vi "GPS PPS Syncronisation.vi"() -> ()   [LabVIEW 2015]
doc: "This template is for the Simple NI-USRP Streaming design, a design that shows the basics of streaming data to and from an NI USRP-294x/295x device. Refer to the block diagram for more information about how to use this template."
uses:
  <instrlib>/niUsrpRio/Config/v1/Host/Public/What to Query for.ctl
  Supporting Files/PPS Source.ctl
  <vilib>/userdefined/Silver/nirio_resource_slv.ctl
  SubVIs/Start Trigger.ctl
  <instrlib>/_niInstr/Register Bus/v0/Host/Public/Register Read Request.ctl
  <instrlib>/niUsrpRio/Config/v1/Host/Private/DB Types.ctl
  <vilib>/Utility/error.llb/DialogType.ctl
  PPS_Global_Var.vi
  Supporting Files/test_sup.vi
  <instrlib>/niUsrpRio/Config/v1/Host/niUsrpRio Config v1 Host.lvlib
  <instrlib>/_niInstr/Register Bus/v0/Host/niInstr Register Bus v0 Host.lvlib
panel:
  out "DaughterB":T1 caption="Daughter Board Name"
  in  "Tab Control 2":enum32{"XY Plot", "Coerced Config"}(tab)
  out "String 2":string
  out "XY Graph":cluster{i32[], dbl[]}[](graph)
  out "generating":bool caption="Generating"
  in  "tx.stop":bool
  out "tx.coerced configurations":T2
  in  "Tab Control":T3(tab)
  out "String":string
  out "PPS Pulse":bool
  in  "?":bool
  out "GPS Lock":bool
  in  "scope":string
  in  "What to Query for":T4=enum."GPS Lock Status"
  in  "PPS Source":T5=enum."gps pps"
  in  "Wait for GPS Lock?":bool=TRUE
  out "Minutes Elapsed (GPS Lock)":dbl
  in  "USRP RIO device":T6="RIO0" caption="USRP RIO Device"
  in  "Which Bitfile":string(combo)="Time"
  in  "Transmitter Config":T8={"rf enable 0"=TRUE, "rf config 0"={"antenna"="TX1", "frequency"=2000000000.0, "lo frequency"=-1.0, "level"=0.0}, "rf enable 1"=FALSE, "rf config 1"={"antenna"="TX1", "frequency"=2000000000.0, "lo frequency"=-1.0, "level"=0.0}, "transfer mode"=enum."Finite", "sample rate"=10000000.0, "number of samples"=8192, "start trigger"=enum."Immediate", "tone frequency"=100000.0} {"tone frequency" format="%#.3pHz"; "sample rate" format="%#.3pS/s"; "rf config 0"."level" format="%#_gdBm"; "rf config 0"."lo frequency" format="%#.3pHz"; "rf config 0"."frequency" format="%#.3pHz"; "rf config 1"."level" format="%#_gdBm"; "rf config 1"."lo frequency" format="%#.3pHz"; "rf config 1"."frequency" format="%#.3pHz"}
  out "RtmLog":string
  out "Error String":string
  in  "Debug":enum32{"Page 1", "Page 2"}(tab)
  out "GPSDO Stability Delay":bool
  out "FPGA Interface Open":bool
  out "USRP Session Status":bool
  out "Executing on FPGA":bool
  out "Target Adr.":T9 {"subsystem" format="%b"; "address" format="%.0b"}
  out "FPGA IO A":bool
  out "Halt: 2":bool
  out "Halt: 1":bool
  out "GPS Lock 2":bool
  out "TKeep Lock":bool
  out "PPS Stable":bool
  out "TkPSP":bool
  out "Which Target?":string
  in  "Interface Method":T10(ring)=enum."Open Dynamic Bitfile"
  out "Time Elapsed":string
  out "FPGA Version":dbl
  out "RIO Version":dbl
  out "Data Clock Rate":dbl
  out "Dautr Clock Rate":dbl
  out "FPGA Interface":dbl
  out "FPGA Board Ver.":dbl
  out "Status":dbl
  in  "Color Box":u32(colorbox)=11842740
  # "Overview"
  # "Aditional Config"
  # "Transmitter Config"
  # "Runtime Log Panel"
  # "Current Errors"
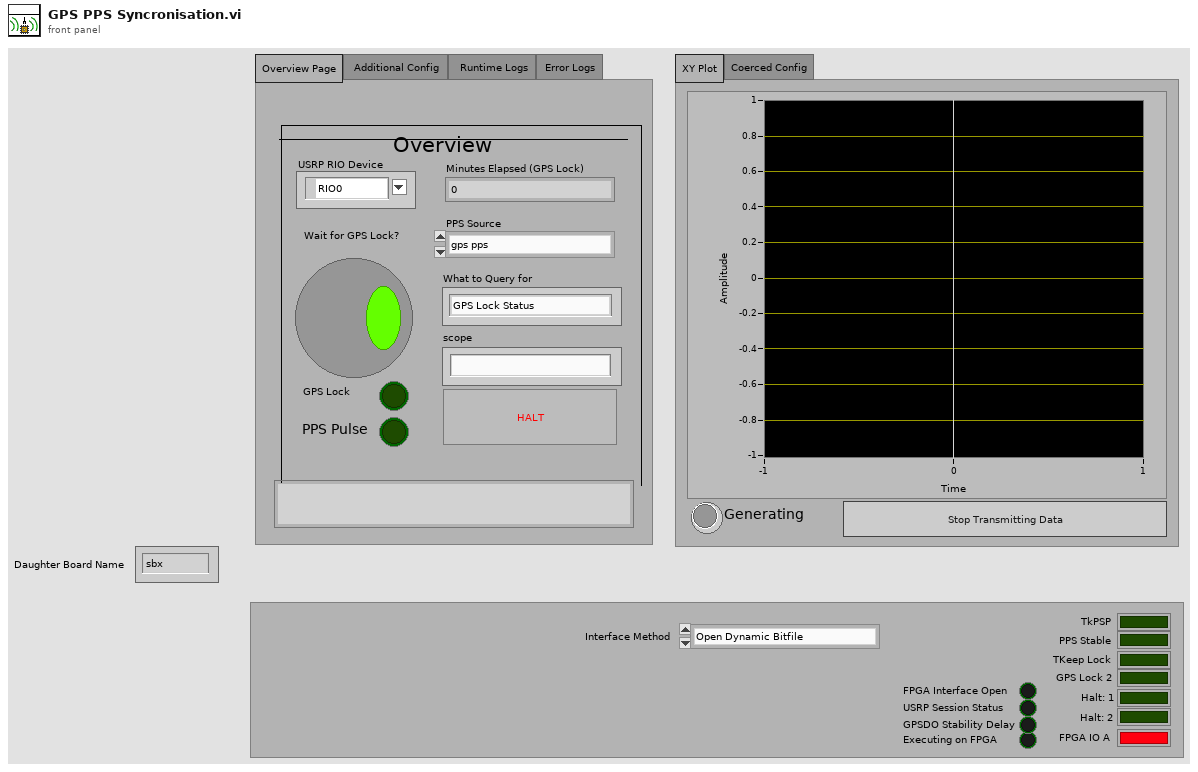
[diagram p1: front panel]
types:
  T1 = typedef "niUsrpRio Config v1 Host.lvlib/DB Types.ctl" = enum16{"sbx", "cbx", "wbx", "unknown"}
  T2 = cluster{"coerced frequencies":dbl[], "coerced lo frequencies":dbl[], "coerced levels":dbl[], "coerced sample rates":dbl[]}
  T3 = enum32{"Overview Page", " Additional Config ", " Runtime Logs ", "Error Logs "}
  T4 = typedef "niUsrpRio Config v1 Host.lvlib/What to Query for.ctl" = enum16{"Clock Chip Lock Status", "Clock Chip Ever Unlocked", "LO Lock Status", "GPS Lock Status", "GPS Ever Unlocked", "DRAM Ready Status", "DAC PLL Lock Status", "DAC Sync Lock Status", "Data Clock PLL Lock Status", "Data Clock PLL Ever Unlocked", "ADC Clock PLL Lock Status", "ADC Clock PLL Ever Unlocked", "ADC Data Valid Status", "ADC Data Ever Invalid"}
  T5 = typedef "PPS Source.ctl" = enum16{"external pps", "gps pps", "internal pps"}
  T6 = typedef "nirio_resource_slv.ctl" = tag
  T7 = typedef "Start Trigger.ctl" = enum8{"Software", "Digital Edge", "Rx Start Trigger", "Tx Start Trigger", "Immediate", "Future Time Event"}
  T8 = cluster{"rf enable 0":bool, "rf config 0":cluster{"antenna":string, "frequency":dbl, "lo frequency":dbl, "level":dbl}, "rf enable 1":bool, "rf config 1":cluster{"antenna":string, "frequency":dbl, "lo frequency":dbl, "level":dbl}, "transfer mode":enum16{"Finite", "Continuous"}, "sample rate":dbl, "number of samples":u32, "start trigger":T7, "tone frequency":dbl}
  T9 = typedef "niInstr Register Bus v0 Host.lvlib/Register Read Request.ctl" = cluster{"subsystem":u8, "address":u16}
  T10 = enum16{"Open FPGA", "Open Dynamic Bitfile", "Daisy Chain"}
  T11 = cluster{"tx config":cluster{"rf enable 0":bool, "rf config 0":cluster{"antenna":string, "frequency":dbl, "lo frequency":dbl, "level":dbl}, "rf enable 1":bool, "rf config 1":cluster{"antenna":string, "frequency":dbl, "lo frequency":dbl, "level":dbl}, "transfer mode":enum16{"Finite", "Continuous"}, "sample rate":dbl, "number of samples":u32, "start trigger":T7, "tone frequency":dbl}, "reference frequency source":string, "tx.enabled channels":string[], "I":i16[], "Q":i16[], "tx.coerced configurations":cluster{"coerced frequencies":dbl[], "coerced lo frequencies":dbl[], "coerced levels":dbl[], "coerced sample rates":dbl[]}}
  T12 = typedef "niUsrpRio Config v1 Host.lvlib/niUsrpRio Session.ctl" = cluster{"FPGA Interface":refnum<k20>, "RIO Interface Number":u32, "Data Clock Rate":u32, "FPGA Data Clock Rate":u32, "Global Settings Register Bus":T13, "Radio 0 Settings Register Bus":T13, "Radio 1 Settings Register Bus":T13, "Radio Settings Bus Semaphore":T14, "DB Queues":T15[], "Characterization Data Valid?":bool, "EEPROM Header":T16, "Device Data Header":T17, "EEPROM Characterization Header":T18, "Characterization Data":T19[], "FPGA Current Version":u32, "FPGA Oldest Compatible Version":u32, "Fixed Logic Current Version":u32, "Fixed Logic Oldest Compatible Version":u32, "FPGA Radio Settings Bus Current Version":u32, "FPGA Radio Settings Bus Oldest Compatible Version":u32, "FPGA Board Config Current Version":u32, "FPGA Board Config Oldest Compatible Version":u32}
  T13 = typedef "niInstr Register Bus v0 Host.lvlib/Register Bus Session.ctl" = refnum<queue>
  T14 = typedef "Semaphore RefNum" = refnum<k1>
  T15 = typedef "niUsrpRio Config v1 Host.lvlib/DB Queue Reference.ctl" = refnum<queue>
  T16 = typedef "niUsrpRio Config v1 Host.lvlib/EEPROM Header.ctl" = cluster{"Checksum":u32, "Product Code":u16, "Hardware Current Version":u16, "Hardware Oldest Compatible Version":u16, "EEPROM Map Current Version":u16, "EEPROM Map Oldest Compatible Version":u16, "User Password":string, "Pointer to Factory Header":u32, "Pointer to User Header":u32, "Recommended Interval":u16, "Number of Reserved Bytes":i32, "Number of Daughterboards":u8, "Daughterboard IDs":u16[], "Daughterboard Serial Numbers":string[]}
  T17 = typedef "niUsrpRio Config v1 Host.lvlib/EEPROM Device Data Header.ctl" = cluster{"Checksum":u32, "Number of Channels":u8, "Number of Gain Settings":u16[], "Pointer to Characterization Data":u32[], "Number of Reserved Bytes":i32, "Number of Frequencies":u16[]}
  T18 = typedef "niUsrpRio Config v1 Host.lvlib/EEPROM Characterization Header.ctl" = cluster{"Checksum":u32, "Date":timestamp, "Temperature":sgl, "Misc. Info":string, "Pointer to Device Data Header":u32, "Number of Reserved Bytes":i32}
  T19 = typedef "niUsrpRio Config v1 Host.lvlib/Characterization Data.ctl" = cluster{"Gains[dB]":dbl[], "Frequencies [Hz]":dbl[], "IQ Imbalance Table":T20[], "Measured Gains[dB]":dbl[][]}
  T20 = typedef "niUsrpRio Config v1 Host.lvlib/IQ Imbalance.ctl" = cluster{"Gain Imbalance [linear]":dbl, "Phase Imbalance [radians]":dbl, "Offset":cdb}
  T21 = typedef "DialogType.ctl" = u16
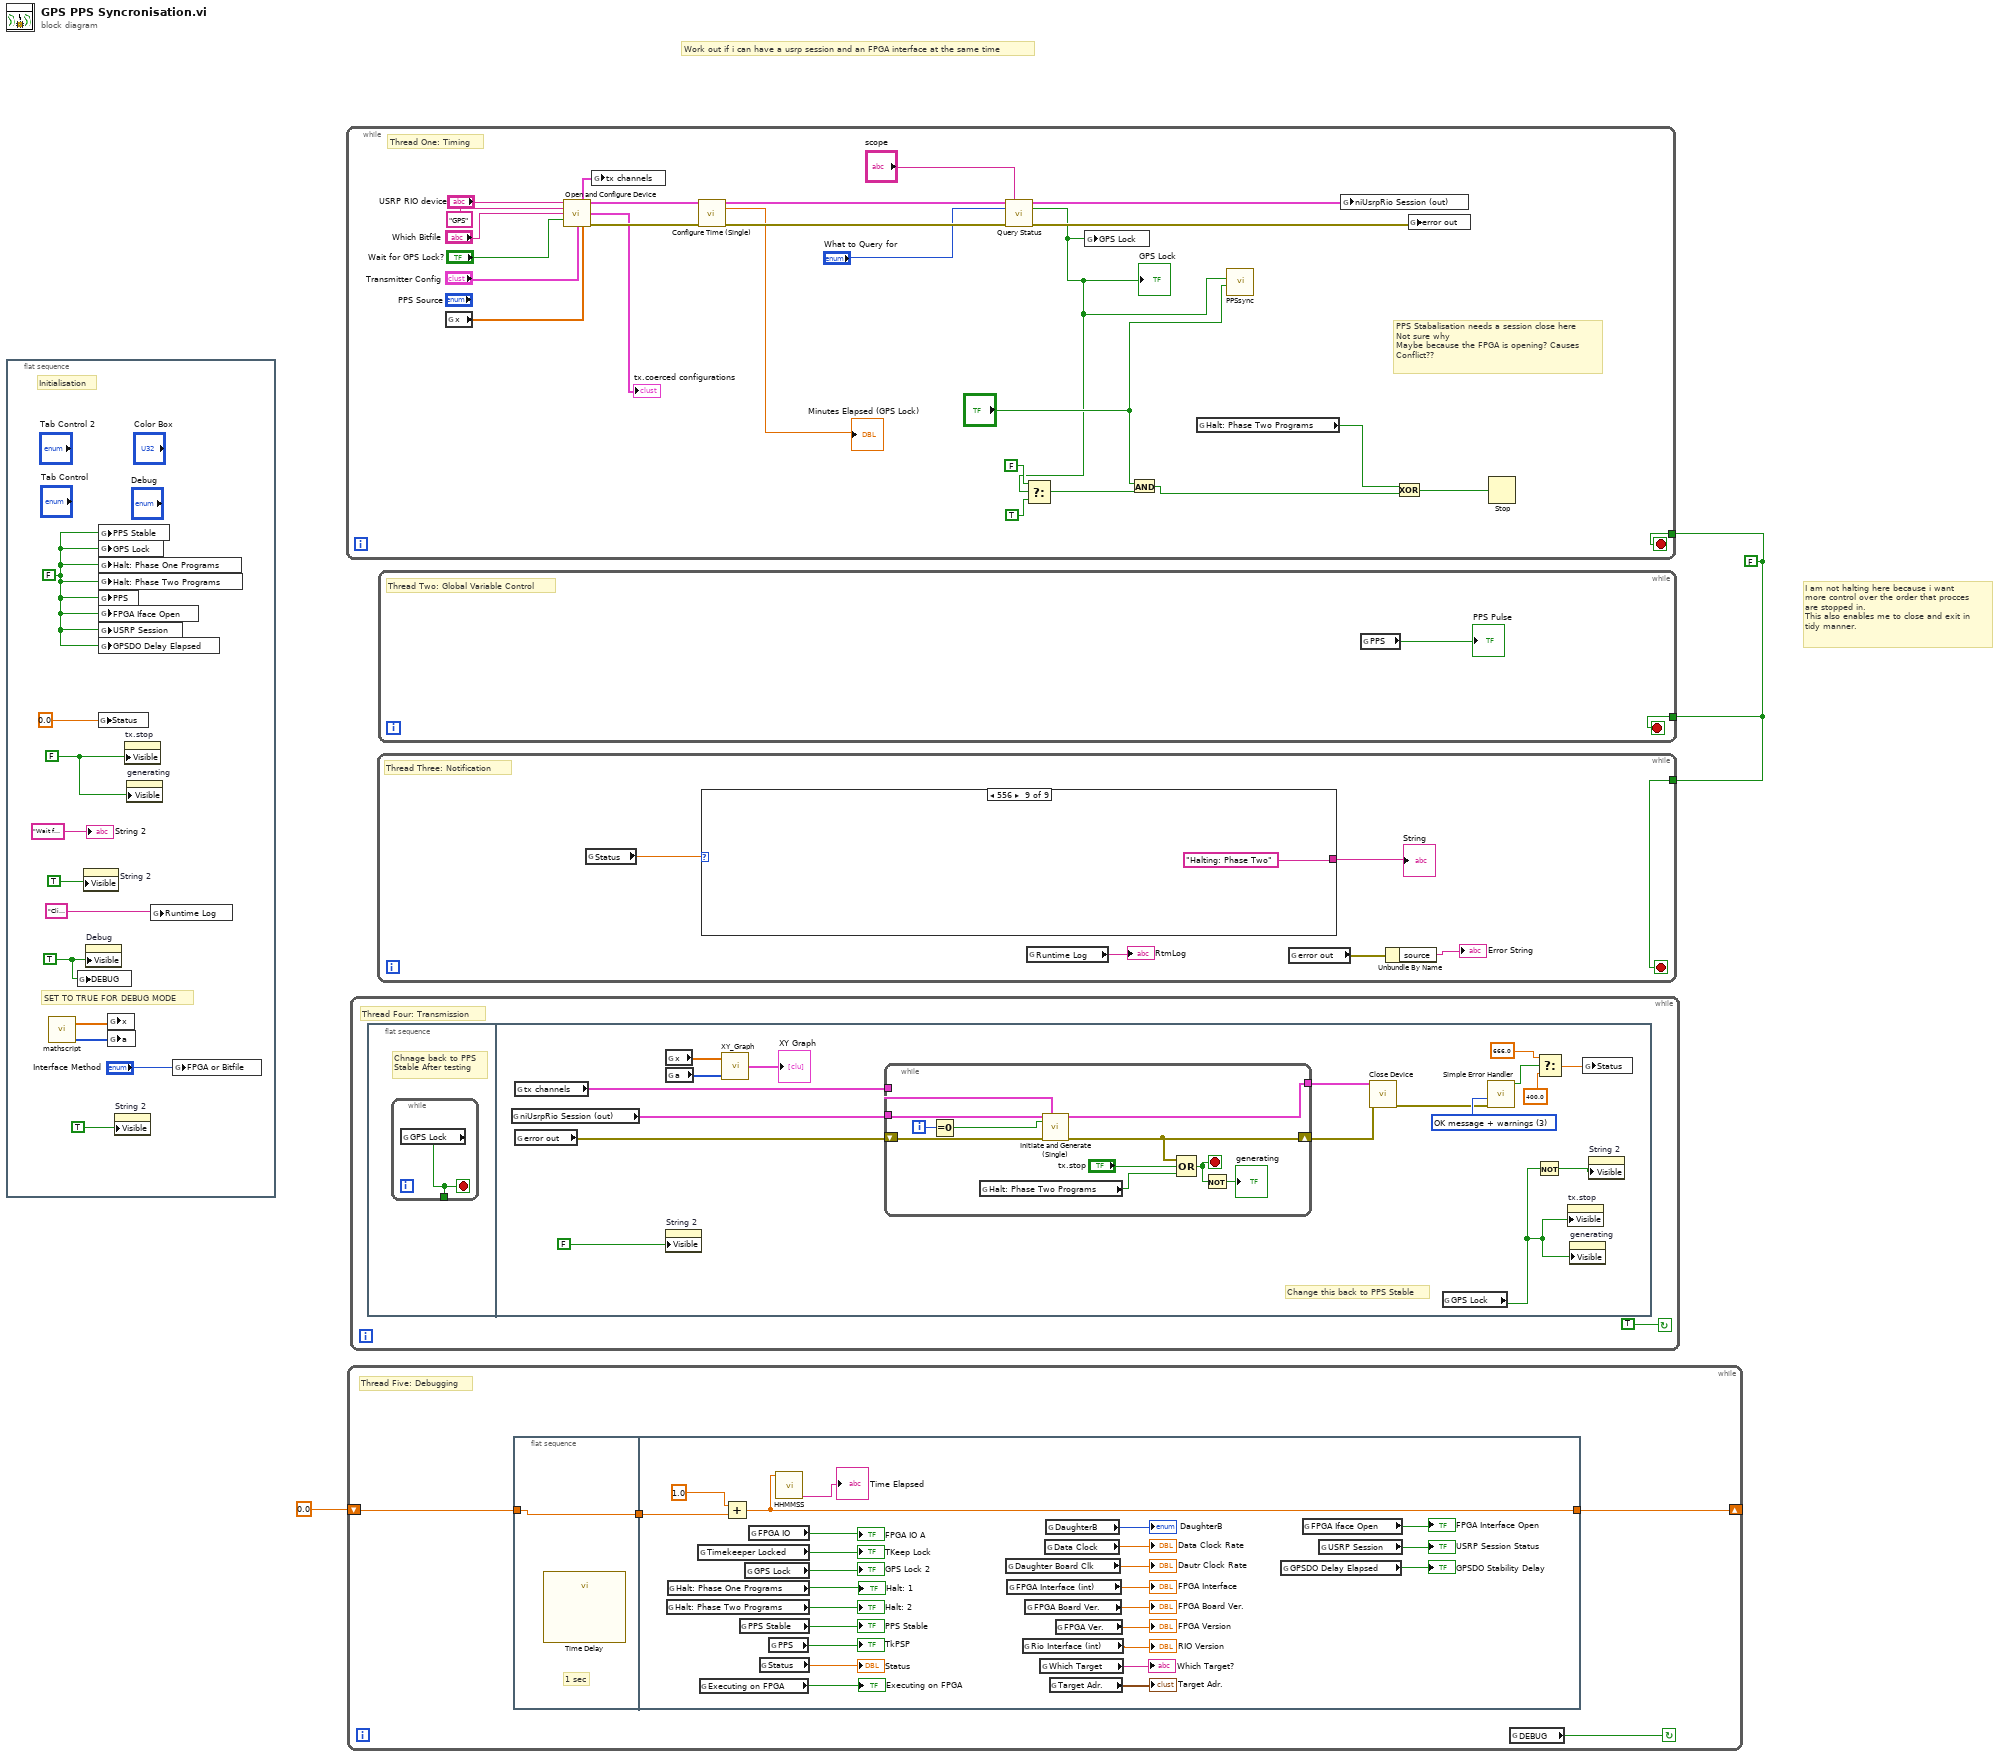
[diagram p0: block diagram]
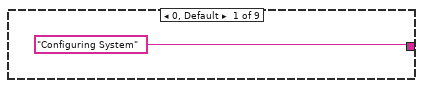
[diagram p2: hidden frame]
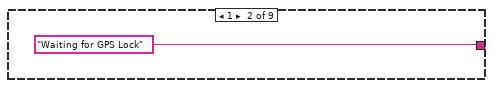
[diagram p3: hidden frame]
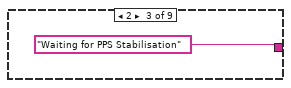
[diagram p4: hidden frame]
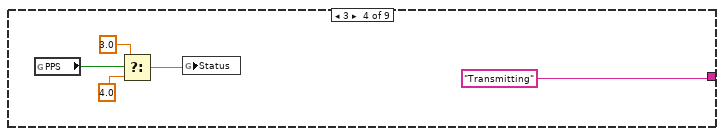
[diagram p5: hidden frame]
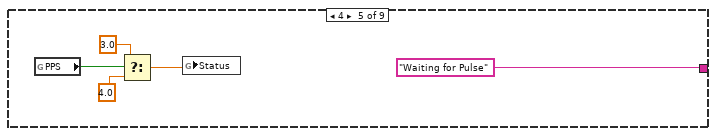
[diagram p6: hidden frame]
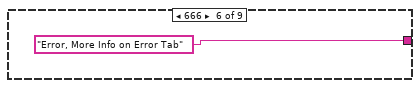
[diagram p7: hidden frame]
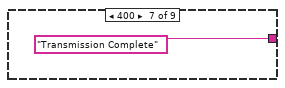
[diagram p8: hidden frame]
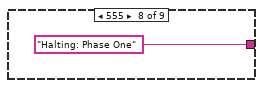
[diagram p9: hidden frame]
diagram:
  w2 = FALSE
  # "Work out if i can have a usrp session and an FPGA interface at the same time"
  # "I am not halting here because i want\nmore control over the order that procces\nare stopped in.\nThis also enables me to close and exit in \ntidy manner."
  n1 = flat-sequence {
    frame #0 {
      w7 = TRUE
      w8 = FALSE
      w5 = FALSE
      # "SET TO TRUE FOR DEBUG MODE"
      # "Initialisation"
      n2 = call "mathscript.vi"() -> ("a"=w11:enum16{""}[], "x"=w12:dbl[])  [unwired: 2 in]
      n3 = global write "PPS_Global_Var.vi" "DEBUG"(w7) -> ()
      n4 = property on="String 2" class="Str"("Visible"=TRUE) -> ()  [unwired: 2 in, 2 out]
      n5 = property on="Debug" class="TabCtl (strict)"("Visible"=w7) -> ()  [unwired: 2 in, 2 out]
      n6 = global write "PPS_Global_Var.vi" "Status"(0.0) -> ()
      n7 = global write "PPS_Global_Var.vi" "PPS Stable"(w5) -> ()
      n8 = global write "PPS_Global_Var.vi" "GPS Lock"(w5) -> ()
      n9 = global write "PPS_Global_Var.vi" "Halt: Phase One Programs"(w5) -> ()
      n10 = global write "PPS_Global_Var.vi" "Halt: Phase Two Programs"(w5) -> ()
      n11 = global write "PPS_Global_Var.vi" "PPS"(w5) -> ()
      n12 = global write "PPS_Global_Var.vi" "FPGA Iface Open"(w5) -> ()
      n13 = global write "PPS_Global_Var.vi" "USRP Session"(w5) -> ()
      n14 = global write "PPS_Global_Var.vi" "GPSDO Delay Elapsed"(w5) -> ()
      n15 = global write "PPS_Global_Var.vi" "x"(w12) -> ()
      n16 = global write "PPS_Global_Var.vi" "a"(w11) -> ()
      n17 = property on="String 2" class="Str"("Visible"=TRUE) -> ()  [unwired: 2 in, 2 out]
      n18 = property on="tx.stop" class="Bool"("Visible"=w8) -> ()  [unwired: 2 in, 2 out]
      n19 = property on="generating" class="Bool (strict)"("Visible"=w8) -> ()  [unwired: 2 in, 2 out]
      n20 = global write "PPS_Global_Var.vi" "Runtime Log"("ClickRun to to Begin") -> ()
      n21 = global write "PPS_Global_Var.vi" "FPGA or Bitfile"("Interface Method") -> ()
      "String 2" <- "Wait for GPS Lock before Transmission Can Begin"
    }
  }
  n22 = while {
    tunnel: w2 -> [w29]
    stop <- w29 stop-if-true
    # "PPS Stabalisation needs a session close here\nNot sure why\nMaybe because the FPGA is opening? Causes\nConflict??"
    # "Thread One: Timing"
    n23 = global read "PPS_Global_Var.vi" "x"() -> (w17:cdb[])
    n24 = call "Open and Configure Device.vi"("USRP RIO Device"="USRP RIO device", "reference frequency source"="GPS", "which bitfile"="Which Bitfile", "Wait for GPS Lock?"="Wait for GPS Lock?", "tx config"="Transmitter Config", "x"=w17) -> ("tx channels"=w18:T11, "niUsrpRio Session (out)"=w38:T12, "tx.coerced configurations"=→"tx.coerced configurations":T2, "error out"=w39:errorcluster)  [unwired: 3 in, 3 out]
    n25 = global write "PPS_Global_Var.vi" "tx channels"(w18) -> ()
    n26 = call "Configure Time (Single).vi"("niUsrpRio Session"=w38, "error in"=w39) -> ("niUsrpRio Session (out)"=w35:T12, "time elapsed"=→"Minutes Elapsed (GPS Lock)":dbl, "error out"=w36:errorcluster)  [unwired: 11 in]
    n27 = call <instrlib>:"Query Status.vi"("niUsrpRio Session"=w35, "scope"="scope", "What to Query for"="What to Query for", "error in"=w36) -> ("niUsrpRio Session (out)"=w16:T12, "Status"=w14:bool, "error out"=w15:errorcluster)  [unwired: 9 in]
    "GPS Lock" <- w14
    n28 = Select(t=FALSE, s=w14, f=TRUE) -> (s? t:f=w32:bool)
    n29 = global write "PPS_Global_Var.vi" "GPS Lock"(w14) -> ()
    n30 = And(x="?", y=w32) -> (x .and. y?=w30:bool)
    n31 = global read "PPS_Global_Var.vi" "Halt: Phase Two Programs"() -> (w28:bool)
    n32 = call "PPSsync.vi"("Halt"="?", "Advance"=w14) -> ()  [unwired: 4 in, 2 out]
    n33 = global write "PPS_Global_Var.vi" "niUsrpRio Session (out)"(w16) -> ()
    n34 = Exclusive Or(1:w30, 2:w28) -> (0:w31:bool)
    n35 = global write "PPS_Global_Var.vi" "error out"(w15) -> ()
    n36 = Stop(stop? (T)=w31) -> ()
  }
  n37 = while {
    shift-right: [w42] -> _
    shift-left: 0.0 -> [w41]
    stop <- w43 continue-if-true
    # "Thread Five: Debugging"
    n38 = flat-sequence {
      tunnel: w41 -> [w44]
      tunnel: [w44] -> w40
      tunnel: [w54] -> w42
      tunnel: w40 -> [w68]
      frame #0 {
        # "1 sec"
        n39 = call "Time Delay"() -> ()  [unwired: 11 in, 1 out]
      }
      frame #1 {
        n40 = global read "PPS_Global_Var.vi" "Halt: Phase Two Programs"() -> (→"Halt: 2":bool)
        n41 = global read "PPS_Global_Var.vi" "Halt: Phase One Programs"() -> (→"Halt: 1":bool)
        n42 = global read "test_sup.vi" "Timekeeper Locked"() -> (→"TKeep Lock":bool)
        n43 = global read "PPS_Global_Var.vi" "Executing on FPGA"() -> (→"Executing on FPGA":bool)
        n44 = Add(x=1.0, y=w68) -> (x+y=w54:dbl)
        n45 = global read "PPS_Global_Var.vi" "PPS Stable"() -> (→"PPS Stable":bool)
        n46 = global read "PPS_Global_Var.vi" "GPS Lock"() -> (→"GPS Lock 2":bool)
        n47 = global read "PPS_Global_Var.vi" "FPGA IO"() -> (→"FPGA IO A":bool)
        n48 = global read "PPS_Global_Var.vi" "Status"() -> (→"Status":dbl)
        n49 = global read "PPS_Global_Var.vi" "PPS"() -> (→"TkPSP":bool)
        n50 = call "HHMMSS.vi"("Time in Seconds"=w54) -> ("HH:MM:SS"=→"Time Elapsed":string)  [unwired: 7 in, 3 out]
        n51 = global read "PPS_Global_Var.vi" "Daughter Board Clk"() -> (→"Dautr Clock Rate":dbl)
        n52 = global read "PPS_Global_Var.vi" "FPGA Interface (int)"() -> (→"FPGA Interface":dbl)
        n53 = global read "PPS_Global_Var.vi" "Rio Interface (int)"() -> (→"RIO Version":dbl)
        n54 = global read "PPS_Global_Var.vi" "FPGA Board Ver."() -> (→"FPGA Board Ver.":dbl)
        n55 = global read "PPS_Global_Var.vi" "Which Target"() -> (→"Which Target?":string)
        n56 = global read "PPS_Global_Var.vi" "Data Clock"() -> (→"Data Clock Rate":dbl)
        n57 = global read "PPS_Global_Var.vi" "DaughterB"() -> (→"DaughterB":T1)
        n58 = global read "PPS_Global_Var.vi" "Target Adr."() -> (→"Target Adr.":T9)
        n59 = global read "PPS_Global_Var.vi" "FPGA Ver."() -> (→"FPGA Version":dbl)
        n60 = global read "PPS_Global_Var.vi" "GPSDO Delay Elapsed"() -> (→"GPSDO Stability Delay":bool)
        n61 = global read "PPS_Global_Var.vi" "FPGA Iface Open"() -> (→"FPGA Interface Open":bool)
        n62 = global read "PPS_Global_Var.vi" "USRP Session"() -> (→"USRP Session Status":bool)
      }
    }
    n63 = global read "PPS_Global_Var.vi" "DEBUG"() -> (w43:bool)
  }
  n64 = while {
    stop <- TRUE continue-if-true
    # "Thread Four: Transmission"
    n65 = flat-sequence {
      frame #0 {
        # "Chnage back to PPS\nStable After testing"
        n66 = while {
          tunnel: [w71] -> _
          stop <- w71 stop-if-true
          n67 = global read "PPS_Global_Var.vi" "GPS Lock"() -> (w71:bool)
        }
      }
      frame #1 {
        w82 = T21 3 items=["no dialog", "OK message", "continue or stop message", "OK message + warnings", "continue/stop + warnings"] ("type of dialog (OK msg:1)")
        # "Change this back to PPS Stable"
        n68 = global read "PPS_Global_Var.vi" "niUsrpRio Session (out)"() -> (w85:T12)
        n69 = global read "PPS_Global_Var.vi" "tx channels"() -> (w84:T11)
        n70 = global read "PPS_Global_Var.vi" "error out"() -> (w76:errorcluster)
        n71 = global read "PPS_Global_Var.vi" "x"() -> (w86:cdb[])
        n72 = global read "PPS_Global_Var.vi" "a"() -> (w87:enum16{""}[])
        n73 = property on="String 2" class="Str"("Visible"=FALSE) -> ()  [unwired: 2 in, 2 out]
        n74 = call "XY_Graph.vi"("a"=w87, "x"=w86) -> ("XY Graph"=→"XY Graph":cluster{i32[], dbl[]}[])
        n75 = while {
          tunnel: w85 -> [w95]
          tunnel: w84 -> [w92]
          tunnel: [w90] -> w77
          shift-right: [w97] -> w78
          shift-left: w76 -> [w94]
          i -> [w93]
          stop <- w96 stop-if-true
          # "Acquire and Fetch a waveform"
          n76 = Equal To 0?(x=w93) -> (x = 0?=w91:bool)
          n77 = global read "PPS_Global_Var.vi" "Halt: Phase Two Programs"() -> (w89:bool)
          n78 = call "Initiate and Generate (Single).vi"("niUsrpRio Session"=w95, "tx channels"=w92, "first iteration"=w91, "error in"=w94) -> ("niUsrpRio Session (out)"=w90:T12, "error out"=w97:errorcluster)  [unwired: 10 in]
          n79 = Compound Arithmetic op=OR(w97, "tx.stop", w89) -> (w96:bool)
          n80 = Not(x=w96) -> (.not. x?=→"generating":bool)
        }
        n81 = call "Close Device.vi"("niUsrpRio Session"=w77, "error in"=w78) -> ("error out"=w81:errorcluster)  [unwired: 13 in]
        n82 = global read "PPS_Global_Var.vi" "GPS Lock"() -> (w83:bool)
        n83 = call <vilib>:"Simple Error Handler.vi"("type of dialog (OK msg:1)"=w82, "error in (no error)"=w81) -> ("error?"=w80:bool)  [unwired: 3 in, 4 out]
        n84 = Not(x=w83) -> (.not. x?=w73:bool)
        n85 = Select(t=666.0, s=w80, f=400.0) -> (s? t:f=w75:dbl)
        n86 = property on="tx.stop" class="Bool"("Visible"=w83) -> ()  [unwired: 2 in, 2 out]
        n87 = property on="generating" class="Bool (strict)"("Visible"=w83) -> ()  [unwired: 2 in, 2 out]
        n88 = global write "PPS_Global_Var.vi" "Status"(w75) -> ()
        n89 = property on="String 2" class="Str"("Visible"=w73) -> ()  [unwired: 2 in, 2 out]
      }
    }
  }
  n90 = while {
    tunnel: w2 -> [w105]
    stop <- w105 stop-if-true
    # "Thread Three: Notification"
    n91 = global read "PPS_Global_Var.vi" "Status"() -> (w104:dbl)
    n92 = case shown="556" w104 {
      tunnel: ["Configuring System" "Waiting for GPS Lock" "Waiting for PPS Stabilisation" "Transmitting" "Waiting for Pulse" "Error, More Info on Error Tab" "Transmission Complete" "Halting: Phase One" "Halting: Phase Two"] -> w103
      frame 0, Default {
      }
      frame 1 {
      }
      frame 2 {
      }
      frame 3 {
        n93 = global read "PPS_Global_Var.vi" "PPS"() -> (w112:bool)
        n94 = Select(t=3.0, s=w112, f=4.0) -> (s? t:f=w111:dbl)
        n95 = global write "PPS_Global_Var.vi" "Status"(w111) -> ()
      }
      frame 4 {
        n96 = global read "PPS_Global_Var.vi" "PPS"() -> (w117:bool)
        n97 = Select(t=3.0, s=w117, f=4.0) -> (s? t:f=w116:dbl)
        n98 = global write "PPS_Global_Var.vi" "Status"(w116) -> ()
      }
      frame 666 {
      }
      frame 400 {
      }
      frame 555 {
      }
      frame 556 {
      }
    }
    "String" <- w103
    n99 = global read "PPS_Global_Var.vi" "Runtime Log"() -> (→"RtmLog":string)
    n100 = global read "PPS_Global_Var.vi" "error out"() -> (w101:errorcluster)
    n101 = Unbundle By Name(w101) -> ("source"=→"Error String":string)
  }
  n102 = while {
    tunnel: w2 -> [w124]
    stop <- w124 stop-if-true
    # "Thread Two: Global Variable Control"
    n103 = global read "PPS_Global_Var.vi" "PPS"() -> (→"PPS Pulse":bool)
  }
